vi "m1m3_logEvent_RejectedAberrationForces.vi"(8 "error in (no error)":errorcluster, 11 "logevent_RejectedAberrationForces_Ctl":T1) -> (0 "error out":errorcluster, 2 "function return":i32, 3 "logevent_RejectedAberrationForces_Ctl out":T1)   [LabVIEW 2016, in "SALLV_m1m3.lvlib"]
doc: "int m1m3_shm_logEvent_RejectedAberrationForcesLV(m1m3_logevent_RejectedAberrationForcesLV *logevent_RejectedAberrationForces_Ctl );"
uses:
  SALLV_m1m3.lvlib
  DataTypes/logevent_RejectedAberrationForces.ctl
  SALLV_m1m3.so
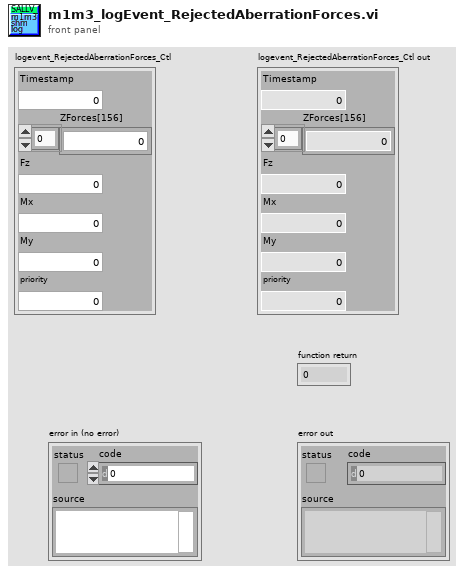
[diagram p1: front panel]
types:
  T1 = typedef "SALLV_m1m3.lvlib/logevent_RejectedAberrationForces.ctl" = cluster{"Timestamp":dbl, "ZForces[156]":sgl[], "Fz":sgl, "Mx":sgl, "My":sgl, "priority":i32}
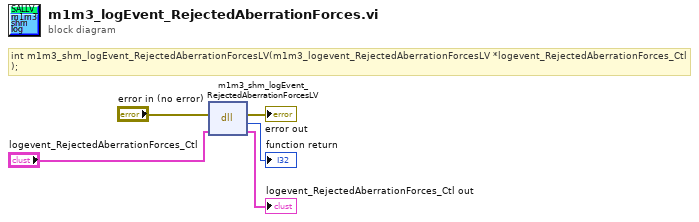
[diagram p0: block diagram]
diagram:
  # "int m1m3_shm_logEvent_RejectedAberrationForcesLV(m1m3_logevent_RejectedAberrationForcesLV *logevent_RejectedAberrationForces_Ctl );"
  n1 = dll-call lib="opt/CODE/SALLV_m1m3/SALLV_m1m3.*" fn="m1m3_shm_logEvent_RejectedAberrationForcesLV"(error in="error in (no error)", "logevent_RejectedAberrationForces_Ctl"="logevent_RejectedAberrationForces_Ctl") -> (error out=→"error out":errorcluster, →"function return":i32, "logevent_RejectedAberrationForces_Ctl"=→"logevent_RejectedAberrationForces_Ctl out":T1)  [unwired: 2 in, 1 out]
